vi "List_Active_Loops.vi"(2 "Alias Table":string[][](array[string]), 3 "Input Sequence":cluster{string, string[], dbl[], dbl}[](array[cluster]), 4 "Loop Count In":cluster{string, "Position":i32}[](array[cluster])) -> (0 "Item List":string[](array[string]), 1 "Loops Out":cluster{string, string[], dbl[], dbl}[](array[cluster]))   [LabVIEW 2011]
doc: "This VI examines the loop count and outputs a formatted array of strings representing all currently active loops."
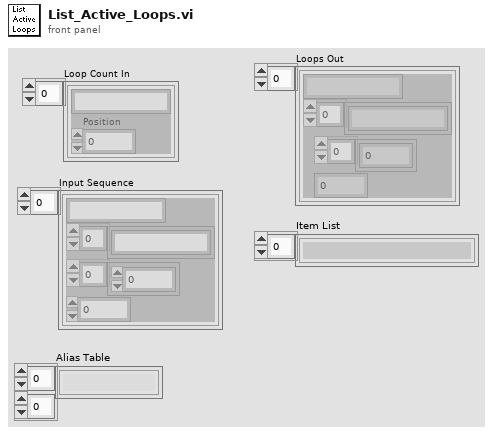
[diagram p1: front panel]
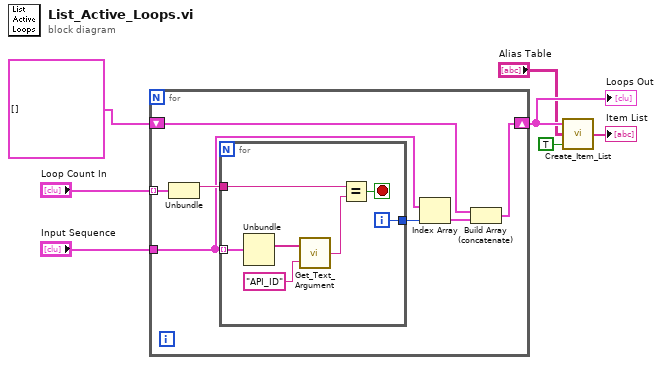
[diagram p0: block diagram]
diagram:
  n1 = for {
    tunnel: "Loop Count In" -> [w14] mode=indexing
    tunnel: "Input Sequence" -> [w11]
    shift-right: [w9] -> w4
    shift-left: cluster{string, string[], dbl[], dbl}[] [] -> [w8]
    n2 = Unbundle(w14) -> (w13:string)  [unwired: 1 out]
    n3 = for {
      tunnel: w11 -> [w21] mode=indexing
      tunnel: w13 -> [w17]
      tunnel: [w15] -> w12
      i -> [w15]
      stop <- w16 stop-if-true
      n4 = Unbundle(w21) -> (w20:string[])  [unwired: 3 out]
      n5 = call "Get_Text_Argument.vi"("Argument"="API_ID", "Argument List"=w20) -> ("Text"=w18:string)
      n6 = Equal?(x=w17, y=w18) -> (x = y?=w16:bool)
    }
    n7 = Index Array(array=w11, index=w12) -> (element=w10:cluster{string, string[], dbl[], dbl})
    n8 = Build Array (concatenate)(w8, w10) -> (w9:cluster{string, string[], dbl[], dbl}[])
  }
  "Loops Out" <- w4
  n9 = call "Create_Item_List.vi"("Running"=TRUE, "Alias Table"="Alias Table", "Sequence"=w4) -> ("Item List"=→"Item List":string[])
